vi "Shock&Dyanamics Laboratory - DROPBEAR_June2022_Rev3.vi"() -> ()   [LabVIEW 2019]
doc: "This example demonstrates how to continuously acquire buffered voltage and thermocouple measurements using a DAQmx device via a single task. In general, DAQmx Create Channel.vi may be called multiple times within a single analog input task if you need to use different channel settings (measurement types, ranges, etc.) across channels on a single device.\n\nFor instructions on how to connect your signals to the DAQ device, refer to your device documentation."
uses:
  LabVIEW DAQ/SubVIs/32CHDAQ - Cases.ctl
  <vilib>/Utility/error.llb/DialogType.ctl
  <vilib>/DAQmx/read.llb/DAQmx Read (Analog 2D DBL NChan NSamp).vi
  <vilib>/DAQmx/read.llb/DAQmx Read (Analog 1D Wfm NChan NSamp).vi
  <vilib>/DAQmx/configure/timing.llb/DAQmx Timing (Sample Clock).vi
  <vilib>/DAQmx/miscellaneous.llb/DAQmx Fill In Error Info.vi
  <vilib>/measure/mamon.llb/Trigger Detection for 1 Channel.vi
  <vilib>/Utility/file.llb/Read Delimited Spreadsheet (DBL).vi
  <resource>/objmgr/daqmx.rc
  <vilib>/measure/NI_MAPro.lvlib
panel:
  out "t2 [ms]":dbl=109.22
  out "t1 [ms]":dbl
  in  "Extensometer Open Volt (V)":dbl=8.5
  in  "Extensometer Gap [mm]":dbl=6.85
  out "Enum":T1(ring)
  in  "Trigger (Yes if on)":bool=TRUE
  out "output cluster 3":T2={{TRUE, "Enable Ch 1"=TRUE, "Enable Ch 2"=TRUE, "Enable Ch 3"=TRUE, "Enable Ch 4"=FALSE, "Enable Ch 5"=FALSE, "Enable Ch 6"=TRUE, "Enable Ch 7"=TRUE, "Enable Ch 8"=FALSE, "Enable Ch 9"=FALSE, "Enable Ch 10"=FALSE, "Enable Ch 11"=FALSE, "Enable Ch 12"=FALSE, "Enable Ch 13"=FALSE, "Enable Ch 14"=FALSE, "Enable Ch 15"=FALSE, "Enable Ch 16"=FALSE, "Enable Ch 17"=FALSE, "Enable Ch 18"=FALSE, "Enable Ch 19"=FALSE, "Enable Ch 20"=FALSE, "Enable Ch 21"=FALSE, "Enable Ch 22"=FALSE, "Enable Ch 23"=FALSE, "Enable Ch 24"=FALSE, "Enable Ch 25"=FALSE, "Enable Ch 26"=FALSE, "Enable Ch 27"=FALSE, "Enable Ch 28"=FALSE, "Enable Ch 29"=FALSE, "Enable Ch 30"=FALSE, "Enable Ch 31"=FALSE}, {"Name (Laser Gate)"="LaserVib", "Name Ch 1"="SG_300_1", "Name Ch 2"="SG_306_b", "Name Ch 3"="Accel", "Name Ch 4"="LowG_accel", "Name Ch 5"="MassDrop", "Name Ch 6"="PinLoc", "Name Ch 7"="Extensometer", "Name Ch 8"="StrainGauge_08_000", "Name Ch 9"="StrainGauge_08_180", "Name Ch 10"="noname", "Name Ch 11"="noname", "Name Ch 12"="noname", "Name Ch 13"="noname", "Name Ch 14"="noname", "Name Ch 15"="noname", "Name Ch 16"="noname", "Name Ch 17"="noname", "Name Ch 18"="noname", "Name Ch 19"="noname", "Name Ch 20"="noname", "Name Ch 21"="noname", "Name Ch 22"="noname", "Name Ch 23"="noname", "Name Ch 24"="noname", "Name Ch 25"="noname", "Name Ch 26"="noname", "Name Ch 27"="noname", "Name Ch 28"="noname", "Name Ch 29"="noname", "Name Ch 30"="noname", "Name Ch 31"="noname"}, {"Physical Channels Ch 0"="PXI1Slot5/ai5", "Physical Channel Ch 1"="PXI1Slot5/ai0", "Physical Channel Ch 2"="PXI1Slot5/ai1", "Physical Channels Ch 3"="PXI1Slot5/ai4", "Physical Channel Ch 4"="PXI1Slot5/ai5", "Physical Channel Ch 5"="PXI1Slot7/ai0", "Physical Channels Ch 6"="PXI1Slot6/ai0", "Physical Channel Ch 7"="PXI1Slot7/ai3", "Physical Channel Ch 8"="PXI1Slot7/ai2", "Physical Channel Ch 9"="PXI1Slot7/ai3", "Physical Channel Ch 10"="PXI1Slot5/ai2", "Physical Channel Ch 11"="PXI1Slot5/ai2", "Physical Channel Ch 12"="PXI1Slot5/ai2", "Physical Channel Ch 13"="PXI1Slot5/ai2", "Physical Channel Ch 14"="PXI1Slot5/ai2", "Physical Channel Ch 15"="PXI1Slot5/ai2", "Physical Channel Ch 16"="PXI1Slot8/ai3", "Physical Channel Ch 17"="PXI1Slot5/ai2", "Physical Channel Ch 18"="PXI1Slot5/ai2", "Physical Channel Ch 19"="PXI1Slot5/ai2", "Physical Channel Ch 20"="PXI1Slot5/ai2", "Physical Channel Ch 21"="PXI1Slot5/ai2", "Physical Channel Ch 22"="PXI1Slot5/ai2", "Physical Channel Ch 23"="PXI1Slot5/ai2", "Physical Channel Ch 24"="PXI1Slot8/ai3", "Physical Channel Ch 25"="PXI1Slot5/ai2", "Physical Channel Ch 26"="PXI1Slot5/ai2", "Physical Channel Ch 27"="PXI1Slot5/ai2", "Physical Channel Ch 28"="PXI1Slot5/ai2", "Physical Channel Ch 29"="PXI1Slot5/ai2", "Physical Channel Ch 30"="PXI1Slot5/ai2", "Physical Channel Ch 31"="PXI1Slot5/ai2"}, {"Voltage Min Ch 0"=-10.0, "Voltage Min Ch 1"=-10.0, "Voltage Min Ch 2"=-10.0, "Voltage Min Ch 3"=-10.0, "Voltage Min Ch 4"=-10.0, "Voltage Min Ch 5"=-10.0, "Voltage Min Ch 6"=-10.0, "Voltage Min Ch 7"=-1.0, "Voltage Min Ch 8"=-10.0, "Voltage Min Ch 9"=-10.0, "Voltage Min Ch 10"=-10.0, "Voltage Min Ch 11"=-10.0, "Voltage Min Ch 12"=-10.0, "Voltage Min Ch 13"=-10.0, "Voltage Min Ch 14"=-10.0, "Voltage Min Ch 15"=-10.0, "Voltage Min Ch 16"=-10.0, "Voltage Min Ch 17"=-10.0, "Voltage Min Ch 18"=-10.0, "Voltage Min Ch 19"=-10.0, "Voltage Min Ch 20"=-10.0, "Voltage Min Ch 21"=-10.0, "Voltage Min Ch 22"=-10.0, "Voltage Min Ch 23"=-10.0, "Voltage Min Ch 24"=-10.0, "Voltage Min Ch 25"=-10.0, "Voltage Min Ch 26"=-10.0, "Voltage Min Ch 27"=-10.0, "Voltage Min Ch 28"=-10.0, "Voltage Min Ch 29"=-10.0, "Voltage Min Ch 30"=-10.0, "Voltage Min Ch 31"=-10.0}, {"Voltage Max Ch 0"=10.0, "Voltage Max Ch 1"=10.0, "Voltage Max Ch 2"=10.0, "Voltage Max Ch 3"=10.0, "Voltage Max Ch 4"=10.0, "Voltage Max Ch 5"=10.0, "Voltage Max  Ch 6"=10.0, "Voltage Max Ch 7"=10.0, "Voltage Max Ch 8"=10.0, "Voltage Max Ch 9"=10.0, "Voltage Max Ch 10"=10.0, "Voltage Max Ch 11"=10.0, "Voltage Max Ch 12"=10.0, "Voltage Max Ch 13"=10.0, "Voltage Max Ch 14"=10.0, "Voltage Max Ch 15"=10.0, "Voltage Max Ch 16"=10.0, "Voltage Max Ch 17"=10.0, "Voltage Max Ch 18"=10.0, "Voltage Max Ch 19"=10.0, "Voltage Max Ch 20"=10.0, "Voltage Max Ch 21"=10.0, "Voltage Max Ch 22"=10.0, "Voltage Max Ch 23"=10.0, "Voltage Max Ch 24"=10.0, "Voltage Max Ch 25"=10.0, "Voltage Max Ch 26"=10.0, "Voltage Max Ch 27"=10.0, "Voltage Max Ch 28"=10.0, "Voltage Max Ch 29"=10.0, "Voltage Max Ch 30"=10.0, "Voltage Max Ch 31"=10.0}, {"Sensitivity 0"=0.5, "Sensitivity 1"=10.0, "Sensitivity 2"=10.0, "Sensitivity 3"=1.0, "Sensitivity 4"=1.0, "Sensitivity 5"=1.0, "Sensitivity 6"=1.0, "Sensitivity 7"=1.0, "Sensitivity 8"=1.0, "Sensitivity 9"=1.0, "Sensitivity 10"=0.2, "Sensitivity 11"=0.2, "Sensitivity 12"=0.2, "Sensitivity 13"=0.2, "Sensitivity 14"=0.2, "Sensitivity 15"=0.2, "Sensitivity 16"=10.0, "Sensitivity 17"=0.2, "Sensitivity 18"=0.2, "Sensitivity 19"=0.2, "Sensitivity 20"=0.2, "Sensitivity 21"=0.2, "Sensitivity 22"=0.2, "Sensitivity 23"=0.2, "Sensitivity 24"=10.0, "Sensitivity 25"=0.2, "Sensitivity 26"=0.2, "Sensitivity 27"=0.2, "Sensitivity 28"=0.2, "Sensitivity 29"=0.2, "Sensitivity 30"=0.2, "Sensitivity 31"=0.2}, {"Sens Fac 0"=enum."V/MU", "Sens Fac 1"=enum."V/MU", "Sens Fac 2"=enum."mV/MU", "Sens Fac 3"=enum."mV/MU", "Sens Fac 4"=enum."mV/MU", "Sens Fac 5"=enum."mV/MU", "Sens Fac 6"=enum."mV/MU", "Sens Fac 7"=enum."mV/MU", "Sens Fac 8"=enum."mV/MU", "Sens Fac 9"=enum."mV/MU", "Sens Fac 10"=enum."uV/MU", "Sens Fac 11"=enum."uV/MU", "Sens Fac 12"=enum."uV/MU", "Sens Fac 13"=enum."uV/MU", "Sens Fac 14"=enum."uV/MU", "Sens Fac 15"=enum."uV/MU", "Sens Fac 16"=enum."mV/MU", "Sens Fac 17"=enum."uV/MU", "Sens Fac 18"=enum."uV/MU", "Sens Fac 19"=enum."uV/MU", "Sens Fac 20"=enum."uV/MU", "Sens Fac 21"=enum."uV/MU", "Sens Fac 22"=enum."uV/MU", "Sens Fac 23"=enum."uV/MU", "Sens Fac 24"=enum."mV/MU", "Sens Fac 25"=enum."uV/MU", "Sens Fac 26"=enum."uV/MU", "Sens Fac 27"=enum."uV/MU", "Sens Fac 28"=enum."uV/MU", "Sens Fac 29"=enum."uV/MU", "Sens Fac 30"=enum."uV/MU", "Sens Fac 31"=enum."uV/MU"}, {"Signal Type 0"=enum."Strain", "Signal Type 1"=enum."Strain", "Signal Type 2"=enum."Strain", "Signal Type 3"=enum."Acceleration", "Signal Type 4"=enum."Voltage", "Signal Type 5"=enum."Voltage", "Signal Type 6"=enum."Voltage", "Signal Type 7"=enum."Voltage", "Signal Type 8"=enum."Strain", "Signal Type 9"=enum."Strain", "Signal Type 10"=enum."Strain", "Signal Type 11"=enum."Strain", "Signal Type 12"=enum."Strain", "Signal Type 13"=enum."Strain", "Signal Type 14"=enum."Strain", "Signal Type 15"=enum."Strain", "Signal Type 16"=enum."Strain", "Signal Type 17"=enum."Strain", "Signal Type 18"=enum."Strain", "Signal Type 19"=enum."Strain", "Signal Type 20"=enum."Strain", "Signal Type 21"=enum."Strain", "Signal Type 22"=enum."Strain", "Signal Type 23"=enum."Strain", "Signal Type 24"=enum."Strain", "Signal Type 25"=enum."Strain", "Signal Type 26"=enum."Strain", "Signal Type 27"=enum."Strain", "Signal Type 28"=enum."Strain", "Signal Type 29"=enum."Strain", "Signal Type 30"=enum."Strain", "Signal Type 31"=enum."Strain"}, {"SG Pair 0"=FALSE, "SG Pair 1"=TRUE, "SG Pair 2"=FALSE, "SG Pair 3"=FALSE, "SG Pair 4"=TRUE, "SG Pair 5"=TRUE, "SG Pair 6"=FALSE, "SG Pair 7"=TRUE, "SG Pair 8"=TRUE, "SG Pair 9"=TRUE, "SG Pair 10"=TRUE, "SG Pair 11"=TRUE, "SG Pair 12"=TRUE, "SG Pair 13"=TRUE, "SG Pair 14"=TRUE, "SG Pair 15"=TRUE, "SG Pair 16"=FALSE, "SG Pair 17"=TRUE, "SG Pair 18"=TRUE, "SG Pair 19"=TRUE, "SG Pair 20"=TRUE, "SG Pair 21"=TRUE, "SG Pair 22"=FALSE, "SG Pair 23"=TRUE, "SG Pair 24"=TRUE, "SG Pair 25"=TRUE, "SG Pair 26"=TRUE, "SG Pair 27"=TRUE, "SG Pair 28"=TRUE, "SG Pair 29"=FALSE, "SG Pair 30"=TRUE, "SG Pair 31"=TRUE}, {"SG Pair Ch 0"=enum."Unpaired", "SG Pair Ch 1"=enum."Ch 2", "SG Pair Ch 2"=enum."Unpaired", "SG Pair Ch 3"=enum."Unpaired", "SG Pair Ch 4"=enum."Unpaired", "SG Pair Ch 5"=enum."Unpaired", "SG Pair Ch 6"=enum."Unpaired", "SG Pair Ch 7"=enum."Unpaired", "SG Pair Ch 8"=enum."Unpaired", "SG Pair Ch 9"=enum."Unpaired", "SG Pair Ch 10"=enum."Unpaired", "SG Pair Ch 11"=enum."Unpaired", "SG Pair Ch 12"=enum."Unpaired", "SG Pair Ch 13"=enum."Unpaired", "SG Pair Ch 14"=enum."Unpaired", "SG Pair Ch 15"=enum."Unpaired", "SG Pair Ch 16"=enum."Unpaired", "SG Pair Ch 17"=enum."Unpaired", "SG Pair Ch 18"=enum."Unpaired", "SG Pair Ch 19"=enum."Unpaired", "SG Pair Ch 20"=enum."Unpaired", "SG Pair Ch 21"=enum."Unpaired", "SG Pair Ch 22"=enum."Unpaired", "SG Pair Ch 23"=enum."Unpaired", "SG Pair Ch 24"=enum."Unpaired", "SG Pair Ch 25"=enum."Unpaired", "SG Pair Ch 26"=enum."Unpaired", "SG Pair Ch 27"=enum."Unpaired", "SG Pair Ch 28"=enum."Unpaired", "SG Pair Ch 29"=enum."Unpaired", "SG Pair Ch 30"=enum."Unpaired", "SG Pair Ch 31"=enum."Unpaired"}, {"PF Condition 0"=TRUE, "PF Condition 1"=FALSE, "PF Condition 2"=FALSE, "PF Condition 3"=FALSE, "PF Condition 4"=TRUE, "PF Condition 5"=TRUE, "PF Condition 6"=TRUE, "PF Condition 7"=TRUE, "PF Condition 8"=TRUE, "PF Condition 9"=TRUE, "PF Condition 10"=FALSE, "PF Condition 11"=FALSE, "PF Condition 12"=FALSE, "PF Condition 13"=FALSE, "PF Condition 14"=FALSE, "PF Condition 15"=FALSE, "PF Condition 16"=TRUE, "PF Condition 17"=FALSE, "PF Condition 18"=FALSE, "PF Condition 19"=FALSE, "PF Condition 20"=FALSE, "PF Condition 21"=FALSE, "PF Condition 22"=FALSE, "PF Condition 23"=FALSE, "PF Condition 24"=TRUE, "PF Condition 25"=FALSE, "PF Condition 26"=FALSE, "PF Condition 27"=FALSE, "PF Condition 28"=FALSE, "PF Condition 29"=FALSE, "PF Condition 30"=FALSE, "PF Condition 31"=FALSE}, {"PF Info"="0.0 0.0 0", "PF Info"="0.0 1.0 0", "PF Info"="0.0 0.0 0", "PF Info"="0.0 0.0 1", "PF Info"="0.0 0.0 2", "PF Info"="0.0 0.0 3", "PF Info"="0.0 0.0 0", "PF Info"="0.0 0.0 1", "PF Info"="0.0 0.0 2", "PF Info"="0.0 0.0 3", "PF Info"="0.0 0.0 0", "PF Info"="0.0 0.0 0", "PF Info"="0.0 0.0 0", "PF Info"="0.0 0.0 0", "PF Info"="0.0 0.0 0", "PF Info"="0.0 0.0 0", "PF Info"="0.0 5.0 3", "PF Info"="0.0 0.0 0", "PF Info"="0.0 0.0 0", "PF Info"="0.0 0.0 0", "PF Info"="0.0 0.0 0", "PF Info"="0.0 0.0 0", "PF Info"="0.0 0.0 0", "PF Info"="0.0 0.0 0", "PF Info"="0.0 5.0 3", "PF Info"="0.0 0.0 0", "PF Info"="0.0 0.0 0", "PF Info"="0.0 0.0 0", "PF Info"="0.0 0.0 0", "PF Info"="0.0 0.0 0", "PF Info"="0.0 0.0 0", "PF Info"="0.0 0.0 0"}}
  in  "output cluster":T2={{TRUE, "Enable Ch 1"=TRUE, "Enable Ch 2"=TRUE, "Enable Ch 3"=TRUE, "Enable Ch 4"=FALSE, "Enable Ch 5"=FALSE, "Enable Ch 6"=TRUE, "Enable Ch 7"=TRUE, "Enable Ch 8"=FALSE, "Enable Ch 9"=FALSE, "Enable Ch 10"=FALSE, "Enable Ch 11"=FALSE, "Enable Ch 12"=FALSE, "Enable Ch 13"=FALSE, "Enable Ch 14"=FALSE, "Enable Ch 15"=FALSE, "Enable Ch 16"=FALSE, "Enable Ch 17"=FALSE, "Enable Ch 18"=FALSE, "Enable Ch 19"=FALSE, "Enable Ch 20"=FALSE, "Enable Ch 21"=FALSE, "Enable Ch 22"=FALSE, "Enable Ch 23"=FALSE, "Enable Ch 24"=FALSE, "Enable Ch 25"=FALSE, "Enable Ch 26"=FALSE, "Enable Ch 27"=FALSE, "Enable Ch 28"=FALSE, "Enable Ch 29"=FALSE, "Enable Ch 30"=FALSE, "Enable Ch 31"=FALSE}, {"Name (Laser Gate)"="LaserVib", "Name Ch 1"="SG_300_1", "Name Ch 2"="SG_306_b", "Name Ch 3"="Accel", "Name Ch 4"="LowG_accel", "Name Ch 5"="MassDrop", "Name Ch 6"="PinLoc", "Name Ch 7"="Extensometer", "Name Ch 8"="StrainGauge_08_000", "Name Ch 9"="StrainGauge_08_180", "Name Ch 10"="noname", "Name Ch 11"="noname", "Name Ch 12"="noname", "Name Ch 13"="noname", "Name Ch 14"="noname", "Name Ch 15"="noname", "Name Ch 16"="noname", "Name Ch 17"="noname", "Name Ch 18"="noname", "Name Ch 19"="noname", "Name Ch 20"="noname", "Name Ch 21"="noname", "Name Ch 22"="noname", "Name Ch 23"="noname", "Name Ch 24"="noname", "Name Ch 25"="noname", "Name Ch 26"="noname", "Name Ch 27"="noname", "Name Ch 28"="noname", "Name Ch 29"="noname", "Name Ch 30"="noname", "Name Ch 31"="noname"}, {"Physical Channels Ch 0"="PXI1Slot5/ai5", "Physical Channel Ch 1"="PXI1Slot5/ai0", "Physical Channel Ch 2"="PXI1Slot5/ai1", "Physical Channels Ch 3"="PXI1Slot5/ai4", "Physical Channel Ch 4"="PXI1Slot5/ai5", "Physical Channel Ch 5"="PXI1Slot7/ai0", "Physical Channels Ch 6"="PXI1Slot6/ai0", "Physical Channel Ch 7"="PXI1Slot7/ai3", "Physical Channel Ch 8"="PXI1Slot7/ai2", "Physical Channel Ch 9"="PXI1Slot7/ai3", "Physical Channel Ch 10"="PXI1Slot5/ai2", "Physical Channel Ch 11"="PXI1Slot5/ai2", "Physical Channel Ch 12"="PXI1Slot5/ai2", "Physical Channel Ch 13"="PXI1Slot5/ai2", "Physical Channel Ch 14"="PXI1Slot5/ai2", "Physical Channel Ch 15"="PXI1Slot5/ai2", "Physical Channel Ch 16"="PXI1Slot8/ai3", "Physical Channel Ch 17"="PXI1Slot5/ai2", "Physical Channel Ch 18"="PXI1Slot5/ai2", "Physical Channel Ch 19"="PXI1Slot5/ai2", "Physical Channel Ch 20"="PXI1Slot5/ai2", "Physical Channel Ch 21"="PXI1Slot5/ai2", "Physical Channel Ch 22"="PXI1Slot5/ai2", "Physical Channel Ch 23"="PXI1Slot5/ai2", "Physical Channel Ch 24"="PXI1Slot8/ai3", "Physical Channel Ch 25"="PXI1Slot5/ai2", "Physical Channel Ch 26"="PXI1Slot5/ai2", "Physical Channel Ch 27"="PXI1Slot5/ai2", "Physical Channel Ch 28"="PXI1Slot5/ai2", "Physical Channel Ch 29"="PXI1Slot5/ai2", "Physical Channel Ch 30"="PXI1Slot5/ai2", "Physical Channel Ch 31"="PXI1Slot5/ai2"}, {"Voltage Min Ch 0"=-10.0, "Voltage Min Ch 1"=-10.0, "Voltage Min Ch 2"=-10.0, "Voltage Min Ch 3"=-10.0, "Voltage Min Ch 4"=-10.0, "Voltage Min Ch 5"=-10.0, "Voltage Min Ch 6"=-10.0, "Voltage Min Ch 7"=-1.0, "Voltage Min Ch 8"=-10.0, "Voltage Min Ch 9"=-10.0, "Voltage Min Ch 10"=-10.0, "Voltage Min Ch 11"=-10.0, "Voltage Min Ch 12"=-10.0, "Voltage Min Ch 13"=-10.0, "Voltage Min Ch 14"=-10.0, "Voltage Min Ch 15"=-10.0, "Voltage Min Ch 16"=-10.0, "Voltage Min Ch 17"=-10.0, "Voltage Min Ch 18"=-10.0, "Voltage Min Ch 19"=-10.0, "Voltage Min Ch 20"=-10.0, "Voltage Min Ch 21"=-10.0, "Voltage Min Ch 22"=-10.0, "Voltage Min Ch 23"=-10.0, "Voltage Min Ch 24"=-10.0, "Voltage Min Ch 25"=-10.0, "Voltage Min Ch 26"=-10.0, "Voltage Min Ch 27"=-10.0, "Voltage Min Ch 28"=-10.0, "Voltage Min Ch 29"=-10.0, "Voltage Min Ch 30"=-10.0, "Voltage Min Ch 31"=-10.0}, {"Voltage Max Ch 0"=10.0, "Voltage Max Ch 1"=10.0, "Voltage Max Ch 2"=10.0, "Voltage Max Ch 3"=10.0, "Voltage Max Ch 4"=10.0, "Voltage Max Ch 5"=10.0, "Voltage Max  Ch 6"=10.0, "Voltage Max Ch 7"=10.0, "Voltage Max Ch 8"=10.0, "Voltage Max Ch 9"=10.0, "Voltage Max Ch 10"=10.0, "Voltage Max Ch 11"=10.0, "Voltage Max Ch 12"=10.0, "Voltage Max Ch 13"=10.0, "Voltage Max Ch 14"=10.0, "Voltage Max Ch 15"=10.0, "Voltage Max Ch 16"=10.0, "Voltage Max Ch 17"=10.0, "Voltage Max Ch 18"=10.0, "Voltage Max Ch 19"=10.0, "Voltage Max Ch 20"=10.0, "Voltage Max Ch 21"=10.0, "Voltage Max Ch 22"=10.0, "Voltage Max Ch 23"=10.0, "Voltage Max Ch 24"=10.0, "Voltage Max Ch 25"=10.0, "Voltage Max Ch 26"=10.0, "Voltage Max Ch 27"=10.0, "Voltage Max Ch 28"=10.0, "Voltage Max Ch 29"=10.0, "Voltage Max Ch 30"=10.0, "Voltage Max Ch 31"=10.0}, {"Sensitivity 0"=0.5, "Sensitivity 1"=10.0, "Sensitivity 2"=10.0, "Sensitivity 3"=1.0, "Sensitivity 4"=1.0, "Sensitivity 5"=1.0, "Sensitivity 6"=1.0, "Sensitivity 7"=1.0, "Sensitivity 8"=1.0, "Sensitivity 9"=1.0, "Sensitivity 10"=0.2, "Sensitivity 11"=0.2, "Sensitivity 12"=0.2, "Sensitivity 13"=0.2, "Sensitivity 14"=0.2, "Sensitivity 15"=0.2, "Sensitivity 16"=10.0, "Sensitivity 17"=0.2, "Sensitivity 18"=0.2, "Sensitivity 19"=0.2, "Sensitivity 20"=0.2, "Sensitivity 21"=0.2, "Sensitivity 22"=0.2, "Sensitivity 23"=0.2, "Sensitivity 24"=10.0, "Sensitivity 25"=0.2, "Sensitivity 26"=0.2, "Sensitivity 27"=0.2, "Sensitivity 28"=0.2, "Sensitivity 29"=0.2, "Sensitivity 30"=0.2, "Sensitivity 31"=0.2}, {"Sens Fac 0"=enum."V/MU", "Sens Fac 1"=enum."V/MU", "Sens Fac 2"=enum."mV/MU", "Sens Fac 3"=enum."mV/MU", "Sens Fac 4"=enum."mV/MU", "Sens Fac 5"=enum."mV/MU", "Sens Fac 6"=enum."mV/MU", "Sens Fac 7"=enum."mV/MU", "Sens Fac 8"=enum."mV/MU", "Sens Fac 9"=enum."mV/MU", "Sens Fac 10"=enum."uV/MU", "Sens Fac 11"=enum."uV/MU", "Sens Fac 12"=enum."uV/MU", "Sens Fac 13"=enum."uV/MU", "Sens Fac 14"=enum."uV/MU", "Sens Fac 15"=enum."uV/MU", "Sens Fac 16"=enum."mV/MU", "Sens Fac 17"=enum."uV/MU", "Sens Fac 18"=enum."uV/MU", "Sens Fac 19"=enum."uV/MU", "Sens Fac 20"=enum."uV/MU", "Sens Fac 21"=enum."uV/MU", "Sens Fac 22"=enum."uV/MU", "Sens Fac 23"=enum."uV/MU", "Sens Fac 24"=enum."mV/MU", "Sens Fac 25"=enum."uV/MU", "Sens Fac 26"=enum."uV/MU", "Sens Fac 27"=enum."uV/MU", "Sens Fac 28"=enum."uV/MU", "Sens Fac 29"=enum."uV/MU", "Sens Fac 30"=enum."uV/MU", "Sens Fac 31"=enum."uV/MU"}, {"Signal Type 0"=enum."Strain", "Signal Type 1"=enum."Strain", "Signal Type 2"=enum."Strain", "Signal Type 3"=enum."Acceleration", "Signal Type 4"=enum."Voltage", "Signal Type 5"=enum."Voltage", "Signal Type 6"=enum."Voltage", "Signal Type 7"=enum."Voltage", "Signal Type 8"=enum."Strain", "Signal Type 9"=enum."Strain", "Signal Type 10"=enum."Strain", "Signal Type 11"=enum."Strain", "Signal Type 12"=enum."Strain", "Signal Type 13"=enum."Strain", "Signal Type 14"=enum."Strain", "Signal Type 15"=enum."Strain", "Signal Type 16"=enum."Strain", "Signal Type 17"=enum."Strain", "Signal Type 18"=enum."Strain", "Signal Type 19"=enum."Strain", "Signal Type 20"=enum."Strain", "Signal Type 21"=enum."Strain", "Signal Type 22"=enum."Strain", "Signal Type 23"=enum."Strain", "Signal Type 24"=enum."Strain", "Signal Type 25"=enum."Strain", "Signal Type 26"=enum."Strain", "Signal Type 27"=enum."Strain", "Signal Type 28"=enum."Strain", "Signal Type 29"=enum."Strain", "Signal Type 30"=enum."Strain", "Signal Type 31"=enum."Strain"}, {"SG Pair 0"=FALSE, "SG Pair 1"=TRUE, "SG Pair 2"=FALSE, "SG Pair 3"=FALSE, "SG Pair 4"=TRUE, "SG Pair 5"=TRUE, "SG Pair 6"=FALSE, "SG Pair 7"=TRUE, "SG Pair 8"=TRUE, "SG Pair 9"=TRUE, "SG Pair 10"=TRUE, "SG Pair 11"=TRUE, "SG Pair 12"=TRUE, "SG Pair 13"=TRUE, "SG Pair 14"=TRUE, "SG Pair 15"=TRUE, "SG Pair 16"=FALSE, "SG Pair 17"=TRUE, "SG Pair 18"=TRUE, "SG Pair 19"=TRUE, "SG Pair 20"=TRUE, "SG Pair 21"=TRUE, "SG Pair 22"=FALSE, "SG Pair 23"=TRUE, "SG Pair 24"=TRUE, "SG Pair 25"=TRUE, "SG Pair 26"=TRUE, "SG Pair 27"=TRUE, "SG Pair 28"=TRUE, "SG Pair 29"=FALSE, "SG Pair 30"=TRUE, "SG Pair 31"=TRUE}, {"SG Pair Ch 0"=enum."Unpaired", "SG Pair Ch 1"=enum."Ch 2", "SG Pair Ch 2"=enum."Unpaired", "SG Pair Ch 3"=enum."Unpaired", "SG Pair Ch 4"=enum."Unpaired", "SG Pair Ch 5"=enum."Unpaired", "SG Pair Ch 6"=enum."Unpaired", "SG Pair Ch 7"=enum."Unpaired", "SG Pair Ch 8"=enum."Unpaired", "SG Pair Ch 9"=enum."Unpaired", "SG Pair Ch 10"=enum."Unpaired", "SG Pair Ch 11"=enum."Unpaired", "SG Pair Ch 12"=enum."Unpaired", "SG Pair Ch 13"=enum."Unpaired", "SG Pair Ch 14"=enum."Unpaired", "SG Pair Ch 15"=enum."Unpaired", "SG Pair Ch 16"=enum."Unpaired", "SG Pair Ch 17"=enum."Unpaired", "SG Pair Ch 18"=enum."Unpaired", "SG Pair Ch 19"=enum."Unpaired", "SG Pair Ch 20"=enum."Unpaired", "SG Pair Ch 21"=enum."Unpaired", "SG Pair Ch 22"=enum."Unpaired", "SG Pair Ch 23"=enum."Unpaired", "SG Pair Ch 24"=enum."Unpaired", "SG Pair Ch 25"=enum."Unpaired", "SG Pair Ch 26"=enum."Unpaired", "SG Pair Ch 27"=enum."Unpaired", "SG Pair Ch 28"=enum."Unpaired", "SG Pair Ch 29"=enum."Unpaired", "SG Pair Ch 30"=enum."Unpaired", "SG Pair Ch 31"=enum."Unpaired"}, {"PF Condition 0"=TRUE, "PF Condition 1"=FALSE, "PF Condition 2"=FALSE, "PF Condition 3"=FALSE, "PF Condition 4"=TRUE, "PF Condition 5"=TRUE, "PF Condition 6"=TRUE, "PF Condition 7"=TRUE, "PF Condition 8"=TRUE, "PF Condition 9"=TRUE, "PF Condition 10"=FALSE, "PF Condition 11"=FALSE, "PF Condition 12"=FALSE, "PF Condition 13"=FALSE, "PF Condition 14"=FALSE, "PF Condition 15"=FALSE, "PF Condition 16"=TRUE, "PF Condition 17"=FALSE, "PF Condition 18"=FALSE, "PF Condition 19"=FALSE, "PF Condition 20"=FALSE, "PF Condition 21"=FALSE, "PF Condition 22"=FALSE, "PF Condition 23"=FALSE, "PF Condition 24"=TRUE, "PF Condition 25"=FALSE, "PF Condition 26"=FALSE, "PF Condition 27"=FALSE, "PF Condition 28"=FALSE, "PF Condition 29"=FALSE, "PF Condition 30"=FALSE, "PF Condition 31"=FALSE}, {"PF Info"="0.0 0.0 0", "PF Info"="0.0 1.0 0", "PF Info"="0.0 0.0 0", "PF Info"="0.0 0.0 1", "PF Info"="0.0 0.0 2", "PF Info"="0.0 0.0 3", "PF Info"="0.0 0.0 0", "PF Info"="0.0 0.0 1", "PF Info"="0.0 0.0 2", "PF Info"="0.0 0.0 3", "PF Info"="0.0 0.0 0", "PF Info"="0.0 0.0 0", "PF Info"="0.0 0.0 0", "PF Info"="0.0 0.0 0", "PF Info"="0.0 0.0 0", "PF Info"="0.0 0.0 0", "PF Info"="0.0 5.0 3", "PF Info"="0.0 0.0 0", "PF Info"="0.0 0.0 0", "PF Info"="0.0 0.0 0", "PF Info"="0.0 0.0 0", "PF Info"="0.0 0.0 0", "PF Info"="0.0 0.0 0", "PF Info"="0.0 0.0 0", "PF Info"="0.0 5.0 3", "PF Info"="0.0 0.0 0", "PF Info"="0.0 0.0 0", "PF Info"="0.0 0.0 0", "PF Info"="0.0 0.0 0", "PF Info"="0.0 0.0 0", "PF Info"="0.0 0.0 0", "PF Info"="0.0 0.0 0"}}
  out "ON/OFF":T3={"Ch 0"=TRUE, "Ch 1"=TRUE, "Ch 2"=TRUE, "Ch 3"=TRUE, "Ch 4"=FALSE, "Ch 5"=FALSE, "Ch 6"=TRUE, "Ch 7"=TRUE, "Ch 8"=FALSE, "Ch 9"=FALSE, "Ch 10"=FALSE, "Ch 11"=FALSE, "Ch 12"=FALSE, "Ch 13"=FALSE, "Ch 14"=FALSE, "Ch 15"=FALSE, "Ch 16"=FALSE, "Ch 17"=FALSE, "Ch 18"=FALSE, "Ch 19"=FALSE, "Ch 20"=FALSE, "Ch 21"=FALSE, "Ch 22"=FALSE, "Ch 23"=FALSE, "Ch 24"=FALSE, "Ch 25"=FALSE, "Ch 26"=FALSE, "Ch 27"=FALSE, "Ch 28"=FALSE, "Ch 29"=FALSE, "Ch 30"=FALSE, "Ch 31"=FALSE}
  out "Signal Type":T4={"Signal Type 0"=enum."Strain", "Signal Type 1"=enum."Strain", "Signal Type 2"=enum."Strain", "Signal Type 3"=enum."Acceleration", "Signal Type 4"=enum."Voltage", "Signal Type 5"=enum."Voltage", "Signal Type 6"=enum."Voltage", "Signal Type 7"=enum."Voltage", "Signal Type 8"=enum."Strain", "Signal Type 9"=enum."Strain", "Signal Type 10"=enum."Strain", "Signal Type 11"=enum."Strain", "Signal Type 12"=enum."Strain", "Signal Type 13"=enum."Strain", "Signal Type 14"=enum."Strain", "Signal Type 15"=enum."Strain", "Signal Type 16"=enum."Strain", "Signal Type 17"=enum."Strain", "Signal Type 18"=enum."Strain", "Signal Type 19"=enum."Strain", "Signal Type 20"=enum."Strain", "Signal Type 21"=enum."Strain", "Signal Type 22"=enum."Strain", "Signal Type 23"=enum."Strain", "Signal Type 24"=enum."Strain", "Signal Type 25"=enum."Strain", "Signal Type 26"=enum."Strain", "Signal Type 27"=enum."Strain", "Signal Type 28"=enum."Strain", "Signal Type 29"=enum."Strain", "Signal Type 30"=enum."Strain", "Signal Type 31"=enum."Strain"}
  in  "Save Data?":bool
  in  "?":enum32{"Trigger Settings", "Continuous"}(tab)
  in  "Timeout (sec)":dbl=3600.0 format="%0.2f"
  out "Striker Velocity (m/s)":dbl
  in  "Programmer Info":string="None"
  in  "Trigger Level (V)":dbl=-0.04
  in  "Sample Rate (Sa/sec)":dbl=50000.0
  in  "Samples per test (Sa)":i32=50000 format="%.0e"
  out "Actual Sample Rate (Sa/sec)":dbl=50000.0 format="%3.1e"
  out "Armed":bool
  out "Triggered":bool
  out "Actual Sample Rate (Sa/sec)":dbl=1000.0 format="%3.1e"
  in  "Sample Rate (Sa/sec)":dbl=1000.0
  in  "Timeout (sec) 3":dbl=10.0 format="%0.2f"
  in  "End Data Recording":bool
  in  "Refresh Rate":dbl=5.0
  out "Load Test Data 2":bool
  in  "Load Test Data":bool
  out "Save Info":T5={"Programmer Info"="None", "Value"=0.0, "Value"=50000.0}
  in  "Save CH Data":bool
  in  "Load CH Data":bool
  in  "Reset SG Pairs":bool=TRUE
  in  "Start Aquisition":bool
  out "Rate Data":waveform(dbl)[](array[waveform])=[{"t0"=timestamp(0 s since 1904-01-01), "dt"=1.0, "Y"=[]}, {"t0"=timestamp(0 s since 1904-01-01), "dt"=1.0, "Y"=[]}, {"t0"=timestamp(0 s since 1904-01-01), "dt"=1.0, "Y"=[]}]
  out "Scaled Data":waveform(dbl)[](array[waveform])=[{"t0"=timestamp(3680017982.3005104 s since 1904-01-01), "dt"=1.9999999999999998e-05, "Y"=array[50000 elements], "attributes"=variant("NI_ChannelName"=variant(string "LaserVib"), "NI_UnitDescription"=variant(string "um/m"))}, {"t0"=timestamp(3680017982.3005104 s since 1904-01-01), "dt"=1.9999999999999998e-05, "Y"=array[50000 elements], "attributes"=variant("NI_ChannelName"=variant(string "SG_300_1"), "NI_UnitDescription"=variant(string "um/m"))}, {"t0"=timestamp(3680017982.3005104 s since 1904-01-01), "dt"=1.9999999999999998e-05, "Y"=array[50000 elements], "attributes"=variant("NI_ChannelName"=variant(string "SG_306_b"), "NI_UnitDescription"=variant(string "um/m"))}, {"t0"=timestamp(3680017982.3005104 s since 1904-01-01), "dt"=1.9999999999999998e-05, "Y"=array[50000 elements], "attributes"=variant("NI_ChannelName"=variant(string "Accel"), "NI_UnitDescription"=variant(string "g"))}, {"t0"=timestamp(3680017982.3005104 s since 1904-01-01), "dt"=1.9999999999999998e-05, "Y"=array[50000 elements], "attributes"=variant("NI_ChannelName"=variant(string "MassDrop"), "NI_UnitDescription"=variant(string "V"))}, {"t0"=timestamp(3680017982.3005104 s since 1904-01-01), "dt"=1.9999999999999998e-05, "Y"=array[50000 elements], "attributes"=variant("NI_ChannelName"=variant(string "PinLoc"), "NI_UnitDescription"=variant(string "V"))}]
  out "Number of Channels":i32=7
  out "Finished Saving Data":bool
  in  "End Program":bool
  in  "View Data":T6(tab)
  out "Raw Data":waveform(dbl)[](graph) caption="Waveform Graph"
  out "Waveform Graph":waveform(dbl)[](graph)=[{"t0"=timestamp(0 s since 1904-01-01), "dt"=0.001, "Y"=array[27200 elements]}, {"t0"=timestamp(0 s since 1904-01-01), "dt"=0.001, "Y"=array[27200 elements]}, {"t0"=timestamp(0 s since 1904-01-01), "dt"=0.001, "Y"=array[27200 elements]}]
  out "Longitudinal Strain":waveform(dbl)[](graph)
  out "Bending Strain":waveform(dbl)[](graph)
  out "Velocity":waveform(dbl)[](graph)
  out "Acceleration":waveform(dbl)[](graph)
  out "Longitudinal Strain Rate":waveform(dbl)[](graph)
  in  "Channel Settings":T7(tab)=enum."= Log File ="
  in  "Sens Fac 0":enum16{"uV/MU", "mV/MU", "V/MU"}(ring)=enum."mV/MU"
  in  "Sensitivity 0":dbl=2000.0
  in  "Physical Channels Ch 0":tag="PXI1Slot5/ai5" caption="Physical Channels"
  in  "Voltage Min Ch 0":dbl=-10.0 caption="Min Value"
  in  "Voltage Max Ch 0":dbl=10.0 caption="Max Value"
  in  "Name (Laser Gate)":string="Low G Accel"
  in  "Signal Type 0":T8(ring) caption="Signal Type"
  in  "PF Condition 0":bool=TRUE caption="PF Condition"
  in  "PF Chassis 0":dbl caption="Chassis" min=0.0 max=7.0 step=1.0 format="%0#2.1g"
  in  "PF Card 0":dbl caption="Card" min=0.0 max=7.0 step=1.0 format="%0#2.1g"
  in  "PF Channel 0":dbl caption="Channel" min=0.0 max=7.0 step=1.0 format="%0#2.1g"
  in  "SG Pair 0":bool caption="Paired"
  in  "SG Pair Ch 0":T9(ring)=enum."Unpaired"
  in  "SG Pair 1":bool=TRUE caption="Paired"
  in  "Sens Fac 1":enum16{"uV/MU", "mV/MU", "V/MU"}(ring)=enum."mV/MU"
  in  "PF Condition 1":bool caption="PF Condition"
  in  "Physical Channel Ch 1":tag="PXI1Slot5/ai0" caption="Physical Channels"
  in  "Voltage Min Ch 1":dbl=-10.0 caption="Min Value"
  in  "Voltage Max Ch 1":dbl=10.0 caption="Max Value"
  in  "Enable Ch 1":bool=TRUE
  in  "Name Ch 1":string="SG_300_a"
  in  "Sensitivity 1":dbl=50.0 caption="Sensitivity 0"
  in  "Signal Type 1":T8(ring)=enum."Strain" caption="Signal Type"
  in  "PF Chassis 1":dbl caption="Chassis" min=0.0 max=7.0 step=1.0 format="%0#2.1g"
